vi "Method.vi"(4 "Bool":refnum<class "Abs_I64 Integer.lvclass">) -> (1 "Result":T1)   [LabVIEW 2021, in "NOT_I64.lvclass"]
uses:
  NOT_I64.lvclass
  Abs_Types/I64 Integer/Abs_I64 Integer.lvclass
  Abs_Type.ctl
  C:/TSA/LV_Abstract/Source/Functions/Support/Function/One Terminal/I64/AbsFunc_One Term_I64.lvclass
  C:/Program Files (x86)/National Instruments/LabVIEW 2021/vi.lib/TSA/Abstract Data Classes/Abs_Types/I64 Integer/Abs_I64 Integer.lvclass
  Support/Function/One Terminal/I64/AbsFunc_One Term_I64.lvclass/AbsFunc_One Term_I64.ctl
  Support/Function/One Terminal/I64/Properties/Write Numeric A.vi
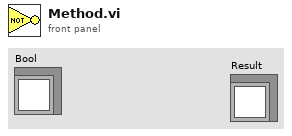
[diagram p1: front panel]
types:
  T1 = typedef "NOT_I64.lvclass/Abs_Type.ctl" = refnum<class "Abs_I64 Integer.lvclass">
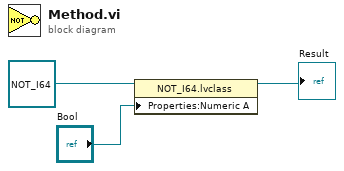
[diagram p0: block diagram]
diagram:
  n1 = property class="NOT_I64.lvclass"(reference=refnum<class "NOT_I64.lvclass"> refnum ("NOT_I64.lvclass"), "Properties:Numeric A"="Bool") -> (reference out=→"Result":refnum<class "NOT_I64.lvclass">)  [unwired: 1 in, 1 out]
